vi "PH_ImageOperator.Beam Analysis.vi"(0 "i ref in":refnum<vi>, 5 "error in (no error)":errorcluster) -> (14 "i ref out":refnum<vi>, 19 "error out":errorcluster)   [LabVIEW 2014, in "PH_ImageOperator.lvlib"]
doc: "This VI does several beam analysis calculations."
uses:
  PH_ImageOperator.lvlib
  <vilib>/vision/NI_Vision_Development_Module.lvlib
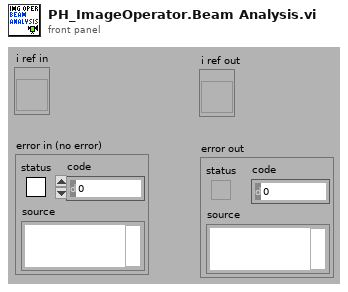
[diagram p1: front panel]
types:
  T1 = typedef "PH_ImageOperator.lvlib/PH_ImageOperator.i attribute.ctl" = cluster{"GUI Refs":cluster{"Delete":refnum<vi>, "Calibration status":refnum<vi>, "BI subtracted":refnum<vi>, "calc Energy":refnum<vi>, "Energy: expected value":refnum<vi>, "Energy: Tolerance":refnum<vi>, "Energy calculated":refnum<vi>, "Energy":refnum<vi>, "calc Beam Anal":refnum<vi>, "Maj Diam 1/esquare":refnum<vi>, "Min Diam 1/esquare":refnum<vi>, "Azi Angle":refnum<vi>, "Min/Maj Diam esquare":refnum<vi>, "Beam analysed":refnum<vi>, "CoG - x":refnum<vi>, "CoG - y":refnum<vi>, "BA: Method":refnum<vi>, "BA: Steps":refnum<vi>, "BA: Factor":refnum<vi>, "calc Traces":refnum<vi>, "Traces: Fit Gauss":refnum<vi>, "Traces calculated":refnum<vi>, "Maj FWHM":refnum<vi>, "Min FWHM":refnum<vi>, "Major Trace":refnum<vi>, "Minor Trace":refnum<vi>, "Maj Fit Order":refnum<vi>, "Min Fit Order":refnum<vi>, "Position calculated":refnum<vi>, "Position":refnum<vi>, "Type":refnum<vi>, "Center":refnum<vi>, "exp - X":refnum<vi>, "exp - Y":refnum<vi>, "Tolerance":refnum<vi>, "f":refnum<vi>, "M":refnum<vi>, "D":refnum<vi>, "q":refnum<vi>, "Dummy Method":refnum<vi>, "Dummy Type":refnum<vi>, "Global On":refnum<vi>, "Traces: No offset":refnum<vi>, "Maj 99%":refnum<vi>, "Min 99%":refnum<vi>, "GUI FF Image":refnum<vi>, "calc Fill Factor":refnum<vi>, "FF calculated":refnum<vi>, "Fill Factor: Filter?":refnum<vi>, "FF: Damage Threshold":refnum<vi>, "FF: Threshold":refnum<vi>, "FF: max allow. Energy":refnum<vi>, "FF: Fillfactor":refnum<vi>, "Calibration data":refnum<vi>}, "List of GUIs":string[], "Calibration":cluster{"Status":T2, "Calibration data":T3, "Calibration Data File":path}, "Final Image":cluster{"BI Subtraction Failure":bool}, "Energy":cluster{"on":bool, "expected value [mJ]":dbl, "Tolerance [%]":dbl, "State":T2, "Energy [mJ]":dbl, "Unit":string, "calculated @":timestamp}, "Beam Analysis":cluster{"on":bool, "Data":T4, "Method":bool, "Steps":i32, "Factor":i32, "ROI":cluster{"Left":i32, "Top":i32, "Right":i32, "Bottom":i32}, "analysed @":timestamp}, "Trace Analysis":cluster{"on":bool, "Fit on":bool, "Maj FWHM":dbl, "Min FWHM":dbl, "Maj Fit Order":i32, "Min Fit Order":i32, "No Offset":bool, "Maj 99%":dbl, "Min 99%":dbl, "Traces":cluster{"XScaleName":string, "Y Scale Minimum":sgl, "Y Scale Maximum":sgl, "X Scale Minimum":sgl, "X Scale Maximum":sgl, "Traces":cluster{"Index":sgl[], "Trace":dbl[]}[]}[], "analysed @":timestamp}, "Position Analysis":cluster{"on":bool, "exp - X":i32, "exp - Y":i32, "focal length [mm]":dbl, "Magnification":dbl, "Delta":dbl, "Theta":dbl, "Tolerance":dbl, "Type":bool, "analysed @":timestamp}, "Fill Factor":cluster{"on":bool, "Filter on?":bool, "Threshold":dbl, "Damage Threshold [J/cm²]":dbl, "Fillfactor":dbl, "Max. allowed Energy [J]":dbl, "calculated @":timestamp}, "Statistician Service ID":i32, "Images":cluster{"Background":T5, "OP":T5, "GUI":T5, "BA: ROI":T5, "Trace: Turn":T5, "FF: Main":T5, "FF: Help":T5, "PSDB: BG":T5, "PSDB: OP":T5, "PSDB: FF":T5}}
  T2 = typedef "PH_StatusHandler.lvlib/PH_StatusHandler.Status.ctl" = i16
  T3 = typedef "PH_ImageCalibrator.lvlib/PH_ImageCalibrator.Calibration Data.ctl" = cluster{"Date":string, "Time":string, "Cam Settings":cluster{"Cam ID":string, "Gain":dbl, "Brightness":dbl, "Shutter":dbl, "Cam Error":bool, "Mode":i32}, "Background Image":cluster{"Image":dbl[][], "Image Error":bool}, "Linear Calibration":cluster{"Calibration Factor":dbl, "not mm or mrad":bool}, "Energy Calibration":cluster{"Calibration Factor":dbl, "no mJ":bool}}
  T4 = typedef "PH_ImageOperator.lvlib/PH_ImageOperator.Beam Analysis Data.ctl" = cluster{"CoG-x":sgl, "CoG-y":sgl, "Maj Dim":dbl, "Min Dim":dbl, "Ellipticity":dbl, "Azimuth Angle [rad]":dbl, "Azi Angle rel to Maj?":bool}
  T5 = typedef "IMAQ Image.ctl" = refnum<image>
  T6 = cluster{"Left":i32, "Top":i32, "Right":i32, "Bottom":i32}
  T7 = cluster{"CoG-x":bool, "CoG-y":bool, "Maj Dim":bool, "Min Dim":bool, "Ellipticity":bool, "Azimuth Angle [rad]":bool, "Azi Angle rel to Maj?":bool}
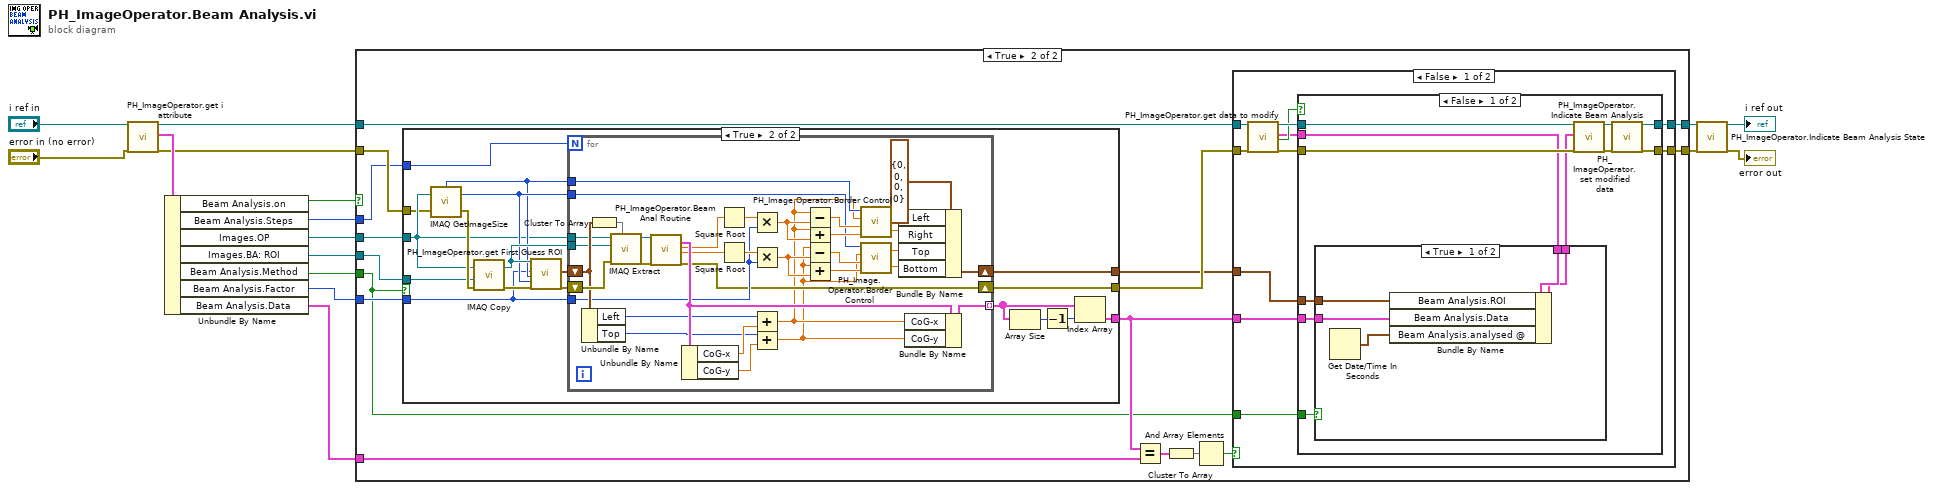
[diagram p0: block diagram]
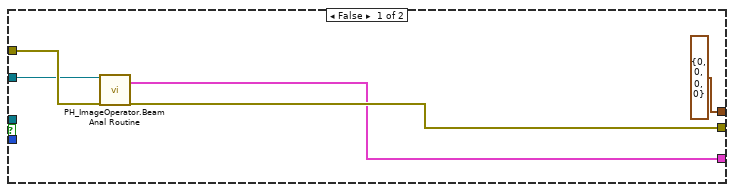
[diagram p3: hidden frame]
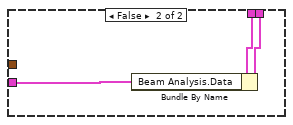
[diagram p4: hidden frame]
diagram:
  n1 = call "PH_ImageOperator.get i attribute.vi"("i ref in"="i ref in", "error in (no error)"="error in (no error)") -> ("i ref out"=w15:refnum<vi>, "i attribute"=w8:T1, "error out"=w7:errorcluster)  [unwired: 15 in]
  n2 = Unbundle By Name(w8) -> ("Beam Analysis.on"=w13:bool, "Beam Analysis.Steps"=w3:i32, "Images.OP"=w2:T5, "Images.BA: ROI"=w1:T5, "Beam Analysis.Method"=w6:bool, "Beam Analysis.Factor"=w4:i32, "Beam Analysis.Data"=w5:T4)
  n3 = case shown="True" w13 {
    tunnel: [w17 w34] -> w9
    tunnel: [w18 w33] -> w11
    tunnel: w7 -> [w17 w30]
    tunnel: w15 -> [w18 w32]
    tunnel: w2 -> [_ w28]
    tunnel: w1 -> [_ w22]
    tunnel: w6 -> [_ w20]
    tunnel: w5 -> [_ w24]
    tunnel: w4 -> [_ w23]
    tunnel: w3 -> [_ w21]
    frame False {
    }
    frame True {
      n4 = case shown="True" w20 {
        tunnel: w30 -> [w39 w46]
        tunnel: [w38 w45] -> w29
        tunnel: w28 -> [w37 w50]
        tunnel: [w36 w44] -> w27
        tunnel: w23 -> [_ w49]
        tunnel: w22 -> [_ w48]
        tunnel: w21 -> [_ w47]
        tunnel: [T6 {"Left"=0, "Top"=0, "Right"=0, "Bottom"=0} ("Rectangle") w40] -> w19
        frame False {
          n5 = call "PH_ImageOperator.Beam Anal Routine.vi"("Image"=w37, "error in (no error)"=w39) -> ("Analysis Data"=w36:T4, "error out"=w38:errorcluster)  [unwired: 13 in, 3 out]
        }
        frame True {
          n6 = call "IMAQ GetImageSize"("Image"=w50, "error in (no error)"=w46) -> ("Y Resolution"=w52:i32, "X Resolution"=w51:i32, "error out"=w53:errorcluster)  [unwired: 2 in]
          n7 = call "IMAQ Copy"("error in (no error)"=w53, "Image Dst"=w48, "Image Src"=w50) -> ("error out"=w57:errorcluster, "Image Dst Out"=w54:T5)  [unwired: 3 in]
          n8 = call "PH_ImageOperator.get First Guess ROI.vi"("Image"=w54, "Factor Std Dev (3)"=w49, "X Resolution"=w51, "Y Resolution"=w52, "error in (no error)"=w57) -> ("First Guess ROI"=w55:T6, "error out"=w56:errorcluster)  [unwired: 13 in]
          n9 = for {
            N: w47 -> [_]
            tunnel: [w77] -> w43 mode=indexing
            tunnel: w50 -> [w76]
            shift-right: [w62] -> w45
            shift-left: w56 -> [w92]
            shift-right: [w58] -> w40
            shift-left: w55 -> [w85]
            tunnel: w54 -> [w75]
            tunnel: w49 -> [w73]
            tunnel: w51 -> [w72]
            tunnel: w52 -> [w67]
            n10 = Unbundle By Name(w85) -> ("Left"=w89:i32, "Top"=w87:i32)
            n11 = Cluster To Array(cluster=w85) -> (array=w88:i32[])
            n12 = call "IMAQ Extract"("Optional Rectangle"=w88, "error in (no error)"=w92, "Image Dst"=w75, "Image Src"=w76) -> ("error out"=w74:errorcluster, "Image Dst Out"=w78:T5)  [unwired: 6 in]
            n13 = call "PH_ImageOperator.Beam Anal Routine.vi"("Image"=w78, "error in (no error)"=w74) -> ("Analysis Data"=w90:T4, "Var-x"=w83:sgl, "Var-y"=w84:sgl, "error out"=w62:errorcluster)  [unwired: 13 in, 1 out]
            n14 = Unbundle By Name(w90) -> ("CoG-x"=w91:sgl, "CoG-y"=w86:sgl)
            n15 = Square Root(x=w83) -> (sqrt(x)=w82:sgl)
            n16 = Square Root(x=w84) -> (sqrt(x)=w81:sgl)
            n17 = Multiply(x=w82, y=w73) -> (x*y=w79:sgl)
            n18 = Multiply(x=w81, y=w73) -> (x*y=w80:sgl)
            n19 = Add(x=w89, y=w91) -> (x+y=w61:sgl)
            n20 = Add(x=w87, y=w86) -> (x+y=w60:sgl)
            n21 = Subtract(x=w61, y=w79) -> (x-y=w71:sgl)
            n22 = Add(x=w61, y=w79) -> (x+y=w69:sgl)
            n23 = Subtract(x=w60, y=w80) -> (x-y=w66:sgl)
            n24 = Add(x=w60, y=w80) -> (x+y=w64:sgl)
            n25 = call "PH_Image.Operator.Border Control.vi"("Calc GreaterBorder"=w69, "Calc Smaller Border"=w71, "CoG"=w61, "Resolution"=w72) -> ("Greater Border"=w68:dbl, "Smaller Border"=w70:dbl)
            n26 = call "PH_Image.Operator.Border Control.vi"("Calc GreaterBorder"=w64, "Calc Smaller Border"=w66, "CoG"=w60, "Resolution"=w67) -> ("Greater Border"=w63:dbl, "Smaller Border"=w65:dbl)
            n27 = Bundle By Name(cluster=T6 {"Left"=0, "Top"=0, "Right"=0, "Bottom"=0} ("Rectangle"), "Left"=w70, "Right"=w68, "Top"=w65, "Bottom"=w63) -> (w58:T6)
            n28 = Bundle By Name(cluster=w90, "CoG-x"=w61, "CoG-y"=w60) -> (w77:T4)
          }
          n29 = Array Size(array=w43) -> (size(s)=w41:i32)
          n30 = Decrement(x=w41) -> (x-1=w42:i32)
          n31 = Index Array(array=w43, index=w42) -> (element=w44:T4)
        }
      }
      n32 = Equal?(x=w27, y=w24) -> (x = y?=w26:T7)
      n33 = Cluster To Array(cluster=w26) -> (array=w25:bool[])
      n34 = And Array Elements(Boolean array=w25) -> (logical AND=w31:bool)
      n35 = case shown="False" w31 {
        tunnel: [w103 w125] -> w34
        tunnel: [w102 w126] -> w33
        tunnel: w32 -> [w97 w126]
        tunnel: w29 -> [w96 w125]
        tunnel: w27 -> [w95 _]
        tunnel: w20 -> [w94 _]
        tunnel: w19 -> [w93 _]
        frame False {
          n36 = call "PH_ImageOperator.get data to modify.vi"("i ref in"=w97, "error in (no error)"=w96) -> ("i ref out"=w101:refnum<vi>, "i attribute"=w98:T1, "timed out"=w99:bool, "error out"=w100:errorcluster)  [unwired: 14 in]
          n37 = case shown="False" w99 {
            tunnel: [w107 w123] -> w103
            tunnel: [w109 w124] -> w102
            tunnel: w101 -> [w114 w124]
            tunnel: w100 -> [w113 w123]
            tunnel: w98 -> [w112 _]
            tunnel: w95 -> [w106 _]
            tunnel: w94 -> [w105 _]
            tunnel: w93 -> [w104 _]
            frame False {
              n38 = case shown="True" w105 {
                tunnel: w112 -> [w119 w122]
                tunnel: [w118 w121] -> w111
                tunnel: w106 -> [w117 w120]
                tunnel: w104 -> [w116 _]
                frame True {
                  n39 = Get Date/Time In Seconds() -> (seconds since 1Jan1904=w115:timestamp)
                  n40 = Bundle By Name(cluster=w119, "Beam Analysis.ROI"=w116, "Beam Analysis.Data"=w117, "Beam Analysis.analysed @"=w115) -> (w118:T1)
                }
                frame False {
                  n41 = Bundle By Name(cluster=w122, "Beam Analysis.Data"=w120) -> (w121:T1)
                }
              }
              n42 = call "PH_ImageOperator.set modified data.vi"("i ref in"=w114, "i attribute"=w111, "error in (no error)"=w113) -> ("i ref out"=w110:refnum<vi>, "error out"=w108:errorcluster)  [unwired: 15 in]
              n43 = call "PH_ImageOperator.Indicate Beam Analysis.vi"("i ref in"=w110, "error in (no error)"=w108) -> ("i ref out"=w109:refnum<vi>, "error out"=w107:errorcluster)  [unwired: 16 in]
            }
            frame True {
            }
          }
        }
        frame True {
        }
      }
    }
  }
  n44 = call "PH_ImageOperator.Indicate Beam Analysis State.vi"("i ref in"=w11, "error in (no error)"=w9) -> ("i ref out"=→"i ref out":refnum<vi>, "error out"=→"error out":errorcluster)  [unwired: 16 in]
